vi "Test Publisher.vi"() -> ()   [LabVIEW 2021]
uses:
  CIFChannels/Typedef/Direction.ctl
  ChannelCommon/typedef/FIFO Config.ctl
  CIF_CIPC_Fifo_U8.lvclass
  ChannelCommon/typedef/TimeStamps.ctl
  <vilib>/CIF Foundation/CIF Utilities/DataTypes/Flatten Unflatten/Flatten U64.vi
  ChannelCommon/ChannelCommon.lvlib
  CIFChannels/CIFChannels.lvclass
panel:
  in  "stop":bool
  out "timed out?":bool
  out "error out":errorcluster
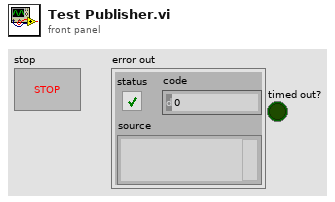
[diagram p1: front panel]
types:
  T1 = typedef "ChannelCommon.lvlib/FIFO Config.ctl" = cluster{"Max Bytes/Msg":u64, "Max Msg/FIFO":u64, "Flags":u64}
  T2 = typedef "CIFChannels.lvclass/Direction.ctl" = enum16{"Publisher", "Subscriber"}
  T3 = typedef "ChannelCommon.lvlib/TimeStamps.ctl" = cluster{"ClockID":u8, "T0":i64, "T_Out":i64}
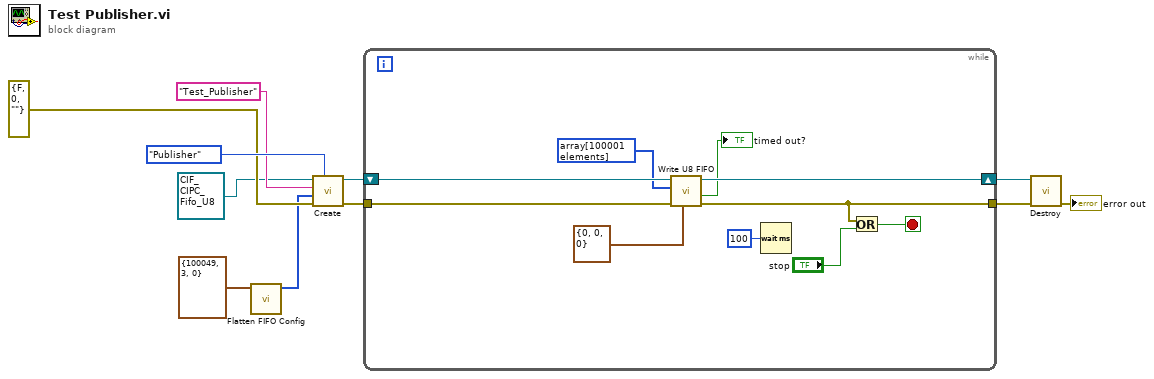
[diagram p0: block diagram]
diagram:
  n1 = call "Flatten FIFO Config.vi"("FIFO Config in"=T1 {"Max Bytes/Msg"=100049, "Max Msg/FIFO"=3, "Flags"=0}) -> ("Flattened FIFO Config"=w2:u8[])  [unwired: 10 in]
  n2 = call-dynamic "Create.vi"("Direction"=Direction."Publisher", "error in (no error)"=errorcluster {"status"=FALSE, "code"=0, "source"=""} ("error out"), "Custom Config Data"=w2, "Name"="Test_Publisher", "CIFFIFO in"=refnum<class "CIF_CIPC_Fifo_U8.lvclass"> refnum ("CIF_CIPC_Fifo_U8.lvclass")) -> ("error out"=w6:errorcluster, "CIFFIFO out"=w7:refnum<class "CIF_CIPC_Fifo_U8.lvclass">)  [unwired: 5 in]
  n3 = while {
    shift-right: [w18] -> w5
    shift-left: w7 -> [w20]
    tunnel: w6 -> [w19]
    tunnel: [w14] -> w4
    stop <- w12 stop-if-true
    n4 = call-dynamic "Write U8 FIFO.vi"("FIFO Timestamps"=T3 {"ClockID"=0, "T0"=0, "T_Out"=0}, "error in (no error)"=w19, "Data in"=u8[] array[100001 elements] ("U8 Data"), "CIFFIFO in"=w20) -> ("error out"=w14:errorcluster, "timed out?"=→"timed out?":bool, "CIFFIFO out"=w18:refnum<class "CIF_CIPC_Fifo_U8.lvclass">)  [unwired: 4 in, 1 out]
    n5 = Wait (ms)(milliseconds to wait=u32 100) -> ()  [unwired: 1 out]
    n6 = Or(x=w14, y="stop") -> (x .or. y?=w12:bool)
  }
  n7 = call-dynamic "Destroy.vi"("error in (no error)"=w4, "CIFFIFO in"=w5) -> ("error out"=→"error out":errorcluster)  [unwired: 8 in, 1 out]
